vi "Purge_FFID_Calib_Gas.vi"(3 "Mode":T5, 5 "Traverse line In":T2 {"Row Duration (mins)" format="%#.1f"; "Row No" min=0; "Trace Gas Concentration (%)" min=0.0 format="%#.2f"; "Emission Rate (l/min)" format="%#.2f"; "Tunnel Speed" format="%#.2f"; "Start X" format="%#.2f"; "Start Y" format="%#.2f"; "Start Z" format="%#.2f"; "End X" format="%#.2f"; "End Y" format="%#.2f"; "End Z" format="%#.2f"; "Averaging time (min)" min=0.0 format="%#.1f"}) -> (0 "Error Message":string, 1 "Status":T1, 2 "Traverse line Out":T2 {"Row Duration (mins)" format="%#.1f"; "Row No" min=0; "Trace Gas Concentration (%)" min=0.0 format="%#.2f"; "Emission Rate (l/min)" format="%#.2f"; "Tunnel Speed" format="%#.2f"; "Start X" format="%#.2f"; "Start Y" format="%#.2f"; "Start Z" format="%#.2f"; "End X" format="%#.2f"; "End Y" format="%#.2f"; "End Z" format="%#.2f"; "Averaging time (min)" min=0.0 format="%#.1f"})   [LabVIEW 2010]
uses:
  Gen Trav/Traverse_cluster.ctl
  Gen Trav/Spacing.ctl
  Controls/Multi_run_mode.ctl
  Controls/User_Specific_mode.ctl
  Gen Trav/Multi_Run_Status.ctl
  ADAM Client/Sub VIs/ADAM Controls/Valco_valve_ph.ctl
panel:
  # "X           Y            Z"
  # "Start"
  # "End"
  # "X           Y            Z"
  # "Start"
  # "End"
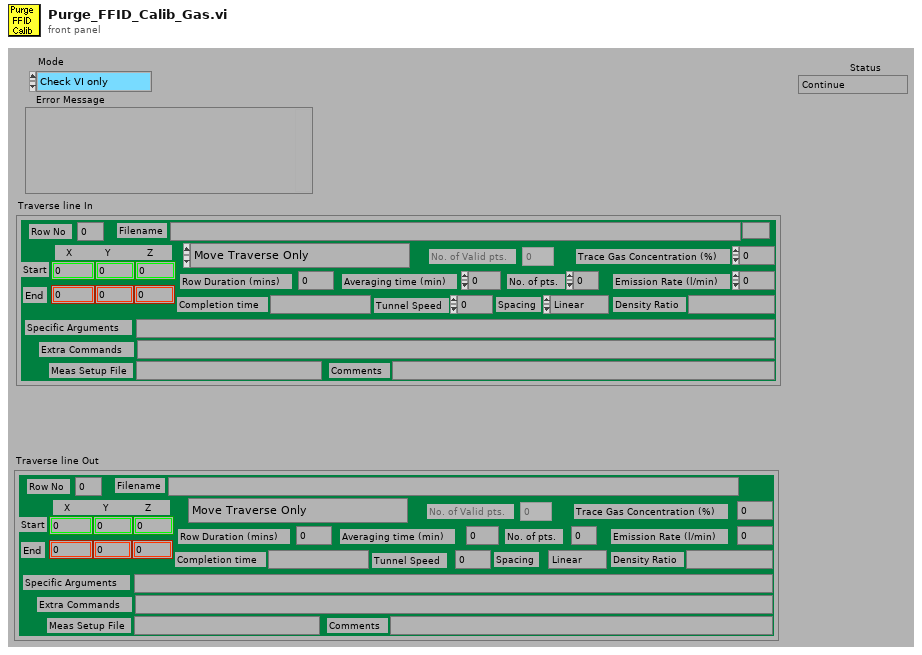
[diagram p1: front panel]
types:
  T1 = typedef "Multi_Run_Status.ctl" = enum16{"Continue", "Jump to Next Point", "Jump to Next Row", "Jump To Fall Back", "Terminate Run"}
  T2 = typedef "Traverse_cluster.ctl" = cluster{"Start X":dbl, "Start Y":dbl, "Start Z":dbl, "End X":dbl, "End Y":dbl, "End Z":dbl, "No. of pts.":i32, "Spacing":T3, "Filename":path, "Tunnel Speed":dbl, "Averaging time (min)":dbl, "Extra Commands":string, "Specific Arguments":string, "Emission Rate (l/min)":dbl, "Trace Gas Concentration (%)":dbl, "Density Ratio":string, "Comments":string, "Row No":i32, "Row Type Selector":T4, "Completion time":string, "Row Duration (mins)":dbl, "No. of Valid pts.":i32, "Meas Setup File":string}
  T3 = typedef "Spacing.ctl" = enum16{"Linear", "Log", "Gauss", "Specified", "N/A"}
  T4 = typedef "Multi_run_mode.ctl" = enum16{"Move Traverse Only", "Set Tunnel Speed Only", "Set Source Only", "Set Measurement Conditions", "Single Measurement", "Vertical Profile", "Lateral Profile", "Longitudinal Profile", "Explore Volume", "Multi-Axis Profile", "Auto Calibrate", "Meas Fast FID Bkgnd", "Check Beam Power", "Scanning Valve Measurement", "Run VI Named:", "Set ADAM Ch", "Wait (minutes)", "Send Message", "Synchronize With:", "Fall Back to this Row", "Turn Off Row Repeating", "Blank Row"}
  T5 = typedef "User_Specific_mode.ctl" = enum16{"Check VI only", "Run VI"}
  T6 = typedef "Valco_valve_ph.ctl" = u16
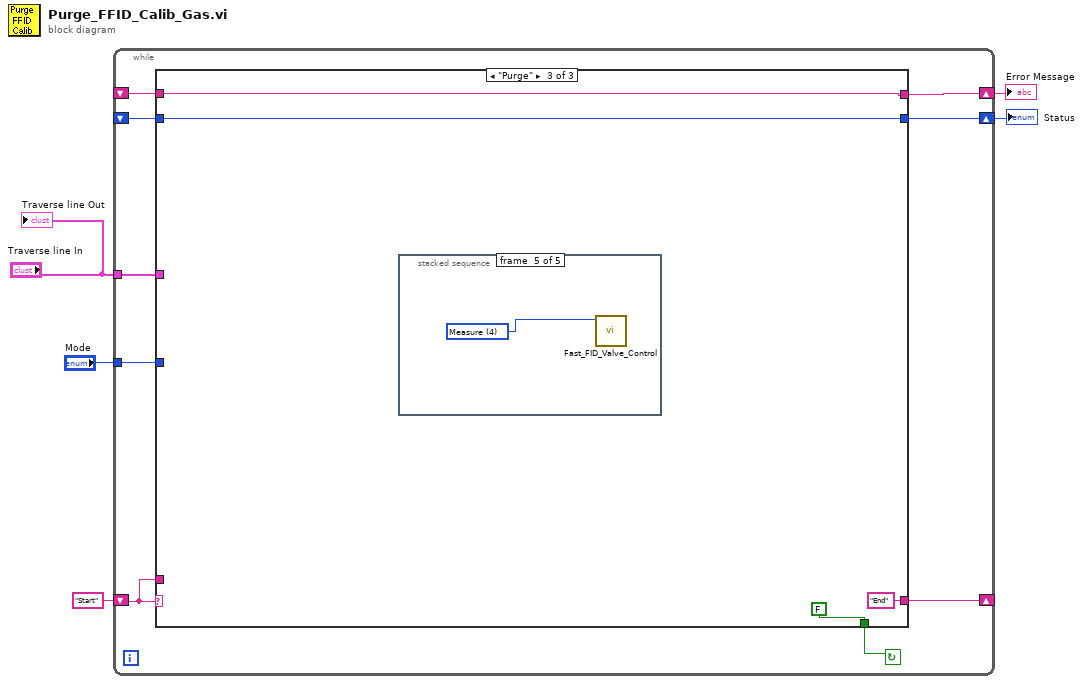
[diagram p0: block diagram]
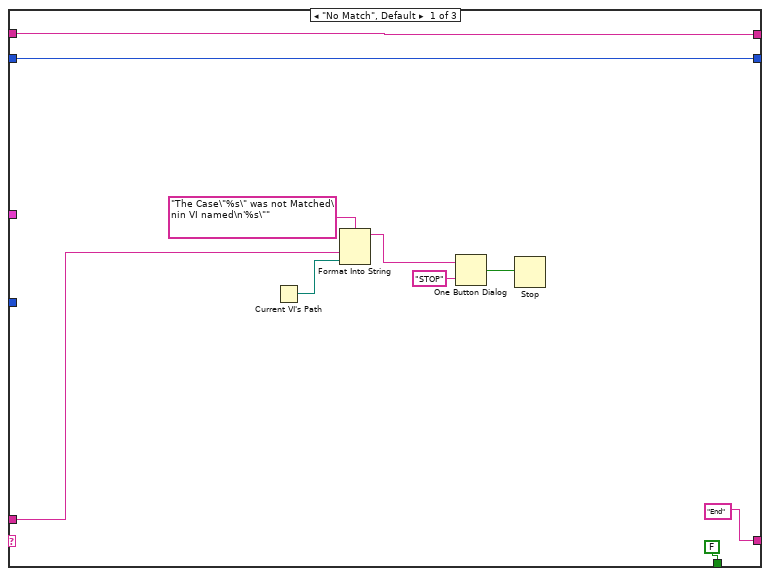
[diagram p2: hidden frame]
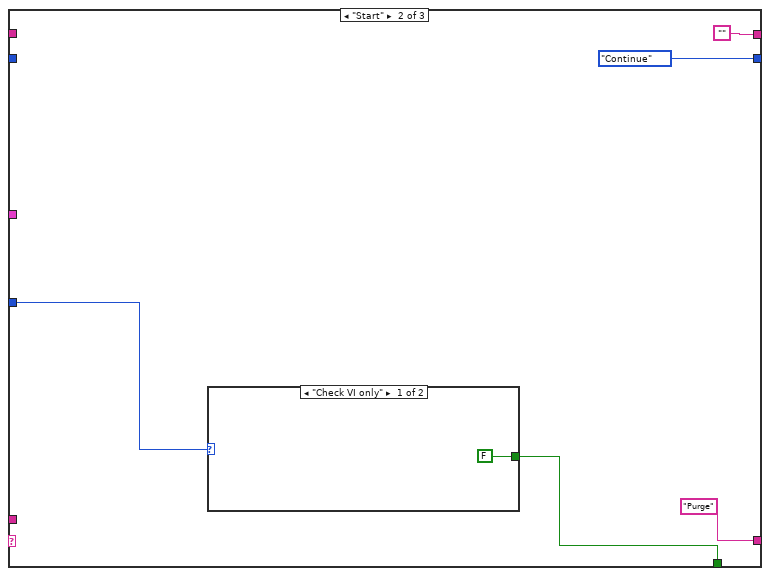
[diagram p3: hidden frame]
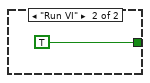
[diagram p4: hidden frame]
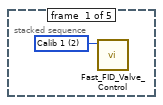
[diagram p5: hidden frame]
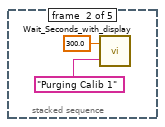
[diagram p6: hidden frame]
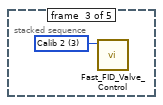
[diagram p7: hidden frame]
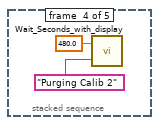
[diagram p8: hidden frame]
diagram:
  n1 = while {
    shift-left: _ -> [w7]
    shift-right: [w6] -> w2
    shift-left: _ -> [w10]
    shift-right: [w8] -> w3
    tunnel: "Traverse line In" -> [w13]
    tunnel: "Mode" -> [w14]
    shift-left: "Start" -> [w9]
    shift-right: [w11] -> _
    stop <- w12 continue-if-true
    n2 = case shown="\"Purge\"" w9 {
      tunnel: w13 -> [_ _ _]
      tunnel: w14 -> [_ w28 _]
      tunnel: [FALSE ("Update Datum Powers?") w27 FALSE ("Update Datum Powers?")] -> w12
      tunnel: ["End" "Purge" "End"] -> w11
      tunnel: w10 -> [w19 _ w32]
      tunnel: [w19 "" w32] -> w8
      tunnel: w9 -> [w16 _ _]
      tunnel: w7 -> [w15 _ w33]
      tunnel: [w15 Multi_Run_Status."Continue" ("Status") w33] -> w6
      frame "No Match", Default {
        n3 = Current VI's Path() -> (path=w20:path)
        n4 = Format Into String(format string="The Case\"%s\" was not Matched\nin VI named\n'%s\"" ("Format String"), w16, w20) -> (resulting string=w23:string)  [unwired: 2 in, 1 out]
        n5 = One Button Dialog(message=w23, button name ("OK")="STOP") -> (true=w21:bool)
        n6 = Stop(stop? (T)=w21) -> ()
      }
      frame "Start" {
        n7 = case shown="\"Check VI only\"" w28 {
          tunnel: [FALSE ("Update Datum Powers?") TRUE ("Update Datum Powers?")] -> w27
          frame "Check VI only" {
          }
          frame "Run VI" {
          }
        }
      }
      frame "Purge" {
        n8 = stacked-sequence {
          frame #0 {
            w36 = T6 2 items=["", "Zero Air", "Calib 1", "Calib 2", "Measure"] ("Requested Position")
            n9 = call "Fast_FID_Valve_Control.vi"("Requested Position"=w36) -> ()  [unwired: 7 out]
          }
          frame #1 {
            n10 = call "Wait_Seconds_with_display.vi"("Message"="Purging Calib 1", "Seconds to wait"=300.0) -> ()  [unwired: 2 out]
          }
          frame #2 {
            w39 = T6 3 items=["", "Zero Air", "Calib 1", "Calib 2", "Measure"] ("Requested Position")
            n11 = call "Fast_FID_Valve_Control.vi"("Requested Position"=w39) -> ()  [unwired: 7 out]
          }
          frame #3 {
            n12 = call "Wait_Seconds_with_display.vi"("Message"="Purging Calib 2", "Seconds to wait"=480.0) -> ()  [unwired: 2 out]
          }
          frame #4 {
            w42 = T6 4 items=["", "Zero Air", "Calib 1", "Calib 2", "Measure"] ("Requested Position")
            n13 = call "Fast_FID_Valve_Control.vi"("Requested Position"=w42) -> ()  [unwired: 7 out]
          }
        }
      }
    }
  }
  "Status" <- w2
  "Error Message" <- w3
  "Traverse line Out" <- "Traverse line In"
